vi "xml_set_use.vi"(0 "target name":string, 1 "in use?":bool, 2 "user":string, 3 "error in (no error)":errorcluster, 4 "XML Path":path=path "D:/Test Management/Farmer/XML/targets.xml") -> (5 "success?":bool, 6 "error out":errorcluster)   [LabVIEW 2011]
uses:
  TargetData.ctl
  <vilib>/xml/Load XML File.vi
  <vilib>/xml/Close Reference(Node).vi
  <vilib>/xml/NI_XML.lvlib
panel:
  in  "Data":T1
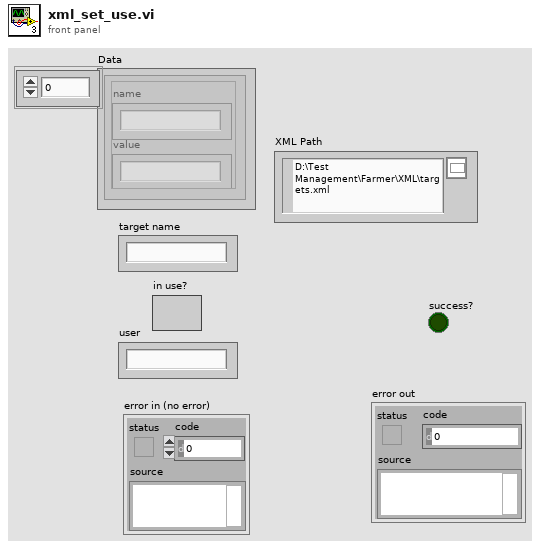
[diagram p1: front panel]
types:
  T1 = typedef "TargetData.ctl" = cluster{"name":string, "value":string}[]
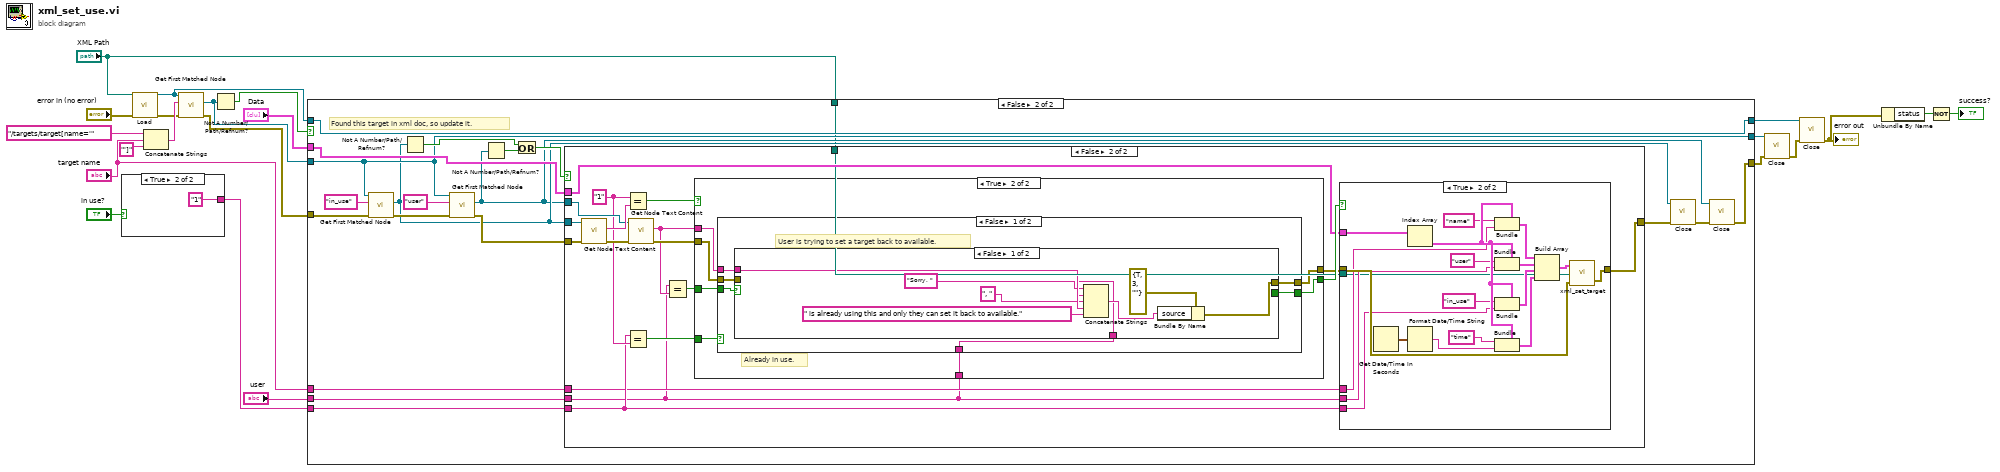
[diagram p0: block diagram]
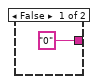
[diagram p2: hidden frame]
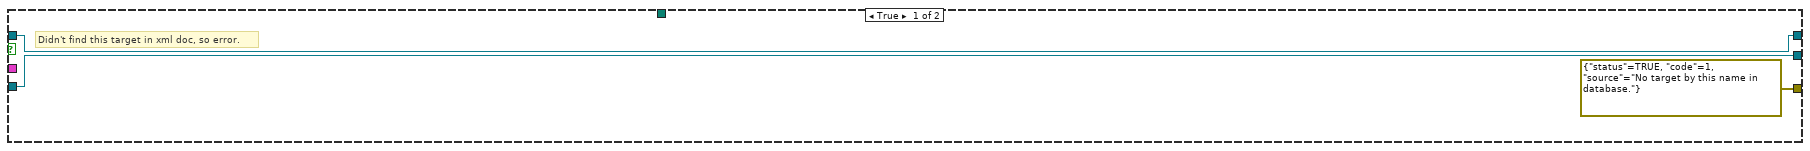
[diagram p3: hidden frame]
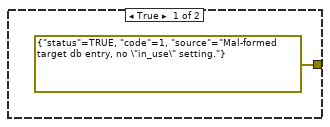
[diagram p4: hidden frame]
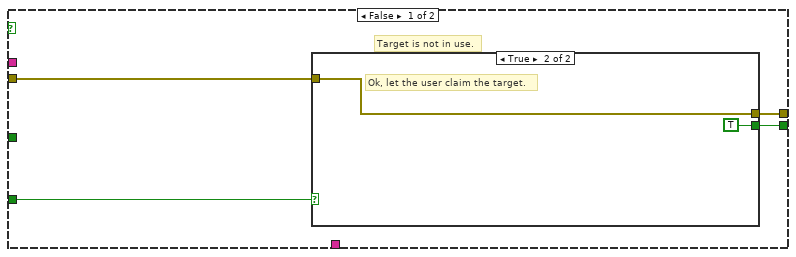
[diagram p6: hidden frame]
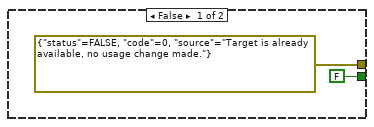
[diagram p7: hidden frame]
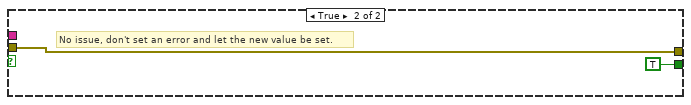
[diagram p8: hidden frame]
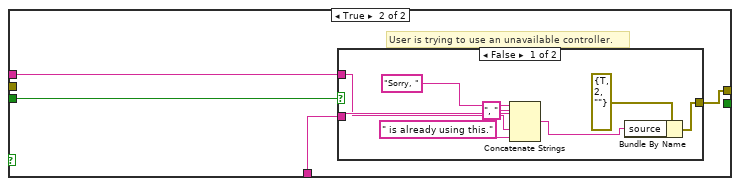
[diagram p9: hidden frame]
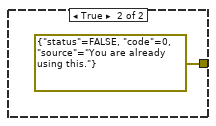
[diagram p10: hidden frame]
diagram:
  n1 = case shown="True" "in use?" {
    tunnel: ["0" "1"] -> w9
    frame False {
    }
    frame True {
    }
  }
  n2 = call-poly <vilib>:"Load.vi"("path to XML document"="XML Path", "error in (no error)"="error in (no error)") -> ("DOM document out"=w3:refnum<k20>, "error out"=w19:errorcluster)  [unwired: 11 in, 1 out]
  n3 = Concatenate Strings("/targets/target[name='", "target name", "']") -> (w20:string)
  n4 = call <vilib>:"Get First Matched Node.vi"("error in (no error)"=w19, "XPath expression"=w20, "node in"=w3) -> ("error out"=w18:errorcluster, "node result"=w15:refnum<k20>)  [unwired: 6 in, 1 out]
  n5 = Not A Number/Path/Refnum?(number/path/refnum=w15) -> (NaN/Path/Refnum?=w17:bool)
  n6 = case shown="False" w17 {
    tunnel: w18 -> [_ w47]
    tunnel: [errorcluster {"status"=TRUE, "code"=1, "source"="No target by this name in database."} ("error out") w31] -> w5
    tunnel: w15 -> [w26 w35]
    tunnel: w9 -> [_ w45]
    tunnel: "user" -> [_ w38]
    tunnel: "Data" -> [_ w37]
    tunnel: "target name" -> [_ w36]
    tunnel: [w26 w35] -> w4
    tunnel: w3 -> [w25 w34]
    tunnel: [w25 w34] -> w2
    tunnel: "XML Path" -> [_ w28]
    frame True {
      # "Didn't find this target in xml doc, so error."
    }
    frame False {
      # "Found this target in xml doc, so update it."
      n7 = call <vilib>:"Get First Matched Node.vi"("error in (no error)"=w47, "XPath expression"="in_use", "node in"=w35) -> ("error out"=w41:errorcluster, "node result"=w30:refnum<k20>)  [unwired: 6 in, 1 out]
      n8 = Not A Number/Path/Refnum?(number/path/refnum=w30) -> (NaN/Path/Refnum?=w44:bool)
      n9 = call <vilib>:"Get First Matched Node.vi"("error in (no error)"=w41, "XPath expression"="user", "node in"=w35) -> ("error out"=w40:errorcluster, "node result"=w29:refnum<k20>)  [unwired: 6 in, 1 out]
      n10 = Not A Number/Path/Refnum?(number/path/refnum=w29) -> (NaN/Path/Refnum?=w42:bool)
      n11 = Or(x=w44, y=w42) -> (x .or. y?=w43:bool)
      n12 = case shown="False" w43 {
        tunnel: [errorcluster {"status"=TRUE, "code"=1, "source"="Mal-formed target db entry, no \"in_use\" setting."} ("error out") w67] -> w32
        tunnel: w30 -> [_ w66]
        tunnel: w40 -> [_ w65]
        tunnel: w45 -> [_ w52]
        tunnel: w29 -> [_ w63]
        tunnel: w38 -> [_ w49]
        tunnel: w37 -> [_ w53]
        tunnel: w36 -> [_ w51]
        tunnel: w28 -> [_ w50]
        frame True {
        }
        frame False {
          w57 = "1" ("x")
          n13 = call <vilib>:"Get Node Text Content.vi"("error in (no error)"=w65, "node in"=w66) -> ("error out"=w62:errorcluster, "node text"=w64:string)  [unwired: 7 in, 1 out]
          n14 = Equal?(x=w57, y=w64) -> (x = y?=w58:bool)
          n15 = Equal?(x=w52, y=w57) -> (x = y?=w56:bool)
          n16 = call <vilib>:"Get Node Text Content.vi"("error in (no error)"=w62, "node in"=w63) -> ("error out"=w61:errorcluster, "node text"=w59:string)  [unwired: 7 in, 1 out]
          n17 = Equal?(x=w49, y=w59) -> (x = y?=w60:bool)
          n18 = case shown="True" w58 {
            tunnel: w61 -> [w90 w98]
            tunnel: w60 -> [_ w102]
            tunnel: [w89 w101] -> w54
            tunnel: w59 -> [_ w100]
            tunnel: w56 -> [w91 w99]
            tunnel: [w88 w97] -> w55
            tunnel: w49 -> [_ w96]
            frame False {
              # "Target is not in use."
              n19 = case shown="True" w91 {
                tunnel: w90 -> [_ w95]
                tunnel: [errorcluster {"status"=FALSE, "code"=0, "source"="Target is already available, no usage change made."} ("error out") w95] -> w89
                tunnel: [FALSE TRUE] -> w88
                frame False {
                }
                frame True {
                  # "Ok, let the user claim the target."
                }
              }
            }
            frame True {
              # "Already in use."
              n20 = case shown="False" w99 {
                tunnel: w102 -> [w108 w122]
                tunnel: [w107 w121] -> w101
                tunnel: w100 -> [w106 w120]
                tunnel: w98 -> [w105 _]
                tunnel: [w104 _] -> w97
                tunnel: w96 -> [w103 w119]
                frame False {
                  # "User is trying to set a target back to available."
                  n21 = case shown="False" w108 {
                    tunnel: [w115 w118] -> w107
                    tunnel: w106 -> [w113 _]
                    tunnel: w105 -> [_ w118]
                    tunnel: [_ TRUE] -> w104
                    tunnel: w103 -> [w110 _]
                    frame False {
                      n22 = Concatenate Strings("Sorry, " ("string"), w110, ", " ("string"), w113, " is already using this and only they can set it back to available." ("string")) -> (w114:string)
                      n23 = Bundle By Name(cluster=errorcluster {"status"=TRUE, "code"=3, "source"=""} ("error in (no error)"), "source"=w114) -> (w115:errorcluster)
                    }
                    frame True {
                      # "No issue, don't set an error and let the new value be set."
                    }
                  }
                }
                frame True {
                  # "User is trying to use an unavailable controller."
                  n24 = case shown="False" w122 {
                    tunnel: [w129 errorcluster {"status"=FALSE, "code"=0, "source"="You are already using this."} ("error in (no error)")] -> w121
                    tunnel: w120 -> [w124 _]
                    tunnel: w119 -> [w125 _]
                    frame False {
                      n25 = Concatenate Strings("Sorry, " ("string"), w125, ", " ("string"), w124, " is already using this." ("string")) -> (w128:string)
                      n26 = Bundle By Name(cluster=errorcluster {"status"=TRUE, "code"=2, "source"=""} ("error in (no error)"), "source"=w128) -> (w129:errorcluster)
                    }
                    frame True {
                    }
                  }
                }
              }
            }
          }
          n27 = case shown="True" w55 {
            tunnel: [w68 w86] -> w67
            tunnel: w54 -> [w68 w87]
            tunnel: w53 -> [_ w83]
            tunnel: w49 -> [_ w75]
            tunnel: w52 -> [_ w74]
            tunnel: w51 -> [_ w73]
            tunnel: w50 -> [_ w69]
            frame False {
            }
            frame True {
              n28 = Get Date/Time In Seconds() -> (seconds since 1Jan1904=w71:timestamp)
              n29 = Index Array(array=w83) -> (element=w82:cluster{"name":string, "value":string})  [unwired: 1 in]
              n30 = Format Date/Time String(seconds (now)=w71) -> (date/time string=w70:string)  [unwired: 2 in]
              n31 = Bundle(cluster=w82, "name"="name", "value"=w73) -> (w84:cluster{"name":string, "value":string})
              n32 = Bundle(cluster=w82, "name"="user", "value"=w75) -> (w81:cluster{"name":string, "value":string})
              n33 = Bundle(cluster=w82, "name"="in_use", "value"=w74) -> (w80:cluster{"name":string, "value":string})
              n34 = Bundle(cluster=w82, "name"="time", "value"=w70) -> (w79:cluster{"name":string, "value":string})
              n35 = Build Array(w84, w81, w80, w79) -> (w85:cluster{"name":string, "value":string}[])
              n36 = call "xml_set_target.vi"("error in (no error)"=w87, "XML Path"=w69, "Data"=w85) -> ("error out"=w86:errorcluster)  [unwired: 1 out]
            }
          }
        }
      }
      n37 = call-poly <vilib>:"Close.vi"("error in (no error)"=w32, "node"=w30) -> ("error out"=w33:errorcluster)  [unwired: 7 in]
      n38 = call-poly <vilib>:"Close.vi"("error in (no error)"=w33, "node"=w29) -> ("error out"=w31:errorcluster)  [unwired: 7 in]
    }
  }
  n39 = call-poly <vilib>:"Close.vi"("error in (no error)"=w5, "node"=w4) -> ("error out"=w16:errorcluster)  [unwired: 7 in]
  n40 = call-poly <vilib>:"Close.vi"("error in (no error)"=w16, "node"=w2) -> ("error out"=w13:errorcluster)  [unwired: 7 in]
  "error out" <- w13
  n41 = Unbundle By Name(w13) -> ("status"=w12:bool)
  n42 = Not(x=w12) -> (.not. x?=→"success?":bool)
